vi "Get Interface Count.vi"(8 "error in (no error)":errorcluster) -> (0 "error out":errorcluster, 3 "count":i32)   [LabVIEW 2017, in "lvwpcap.lvlib"]
uses:
  lvwpcap.lvlib
  LVpcap.dll
panel:
  # "Select Help»Show Context Help and move the cursor over the VI icon to display help for this VI."
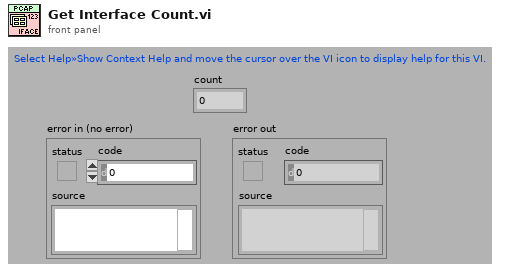
[diagram p1: front panel]
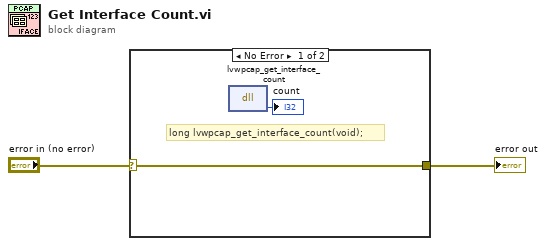
[diagram p0: block diagram]
diagram:
  n1 = case shown="No Error" "error in (no error)" {
    selector: "error in (no error)" -> [w3 w5]
    tunnel: [w3 w5] -> w1
    frame No Error {
      # "long lvwpcap_get_interface_count(void);"
      n2 = dll-call lib="C:/Users/Michaello/Desktop/MGR NOWEEEEEEEEEEEEEE/MR PROFINET 2017/Lib/WinPcap/LVpcap.dll" fn="lvwpcap_get_interface_count"() -> ("return type"=→"count":i32)  [unwired: 3 in, 2 out]
    }
    frame Error {
    }
  }
  "error out" <- w1
